vi "PicoScope6000AWG.vi"(6 "Arbitrary Waveform Settings":T1 {"Index Mode" items=["Single", "Dual", "Quad"]}, 7 "Standard Waveform Settings":T2 {"Start Frequency (Hz)" min=1 max=1000000}, 8 "error in":errorcluster, 9 "General AWG Settings":T3 {"White Noise/PRBS" items=["Normal", "White Noise", "PRBS"]; "Trigger Source" items=["None", "Scope Trigger", "Aux. In", "Ext. In", "Software Trigger"]; "Trigger Type" items=["Rising", "Falling", "Gate High", "Gate Low"]; "Sweep Type" items=["Up", "Down", "Up-Down", "Down-Up"]; "Wave Type" items=["Sine", "Square", "Triangle", "Ramp Up", "Ramp Down", "Sinc", "Gaussian", "Half Sine", "DC", "Arbitrary"]}, 11 "Handle In":i16) -> (0 "error out":errorcluster, 1 "Arbitrary\nWaveform Graph":i16[](graph), 2 "Trigger Source Out":u32, 3 "Handle Out":i16)   [LabVIEW 2009]
doc: "This VI can be used to control the arbitrary waveform generator. Standard waveforms can be selected or arbitrary waveform can be selected under 'Wave Type'. There are three settings clusters: general settings that apply to both arbitrary and standard waveforms, settings that apply only to standard waveforms and settings that apply only to arbitrary waveforms. It is not necessary to connect all of these clusters if only using arbitrary waveforms or only using standard waveforms are required.\n\nWhen selecting arbitrary waveform, it is necessary to specify a text file containing the wave form. This text file should have a single value on each line in the range -1 to 1. For further information on the settings, see descriptions of ps3000aSetSigGenBuiltIn and ps3000aSetSigGenArbitrary."
uses:
  ps6000.dll
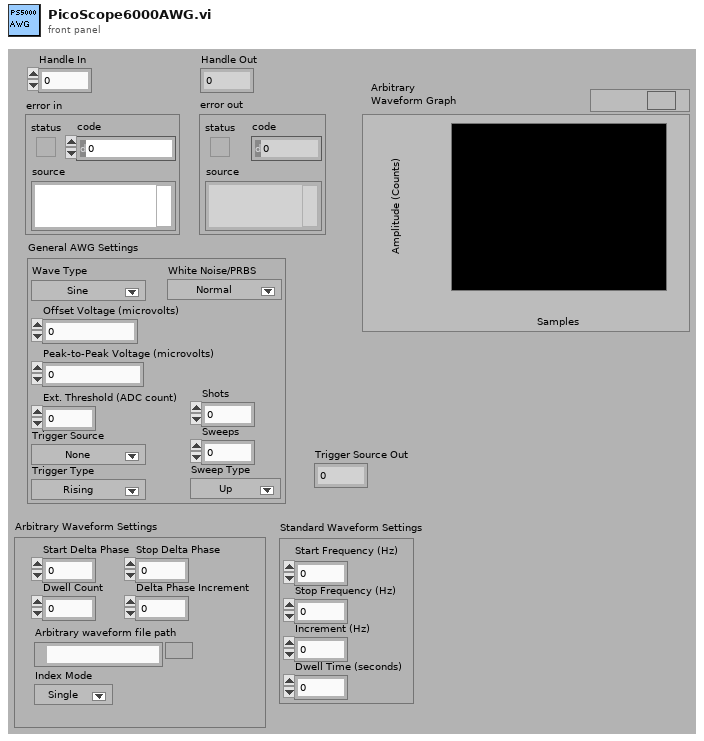
[diagram p1: front panel]
types:
  T1 = cluster{"Arbirary waveform file path":path, "Start Delta Phase":u32, "Index Mode":i32, "Stop Delta Phase":u32, "Delta Phase Increment":u32, "Dwell Count":u32}
  T2 = cluster{"Start Frequency (Hz)":sgl, "Stop Frequency (Hz)":sgl, "Increment (Hz)":sgl, "Dwell Time (seconds)":sgl}
  T3 = cluster{"Peak-to-Peak Voltage (microvolts)":u32, "Offset Voltage (microvolts)":i32, "Wave Type":u32, "Sweep Type":u32, "Shots":u32, "Sweeps":u32, "Trigger Type":u32, "Trigger Source":u32, "Ext. Threshold (ADC count)":i16, "White Noise/PRBS":u32}
  T4 = cluster{"status":bool, "code":u32, "source":string}
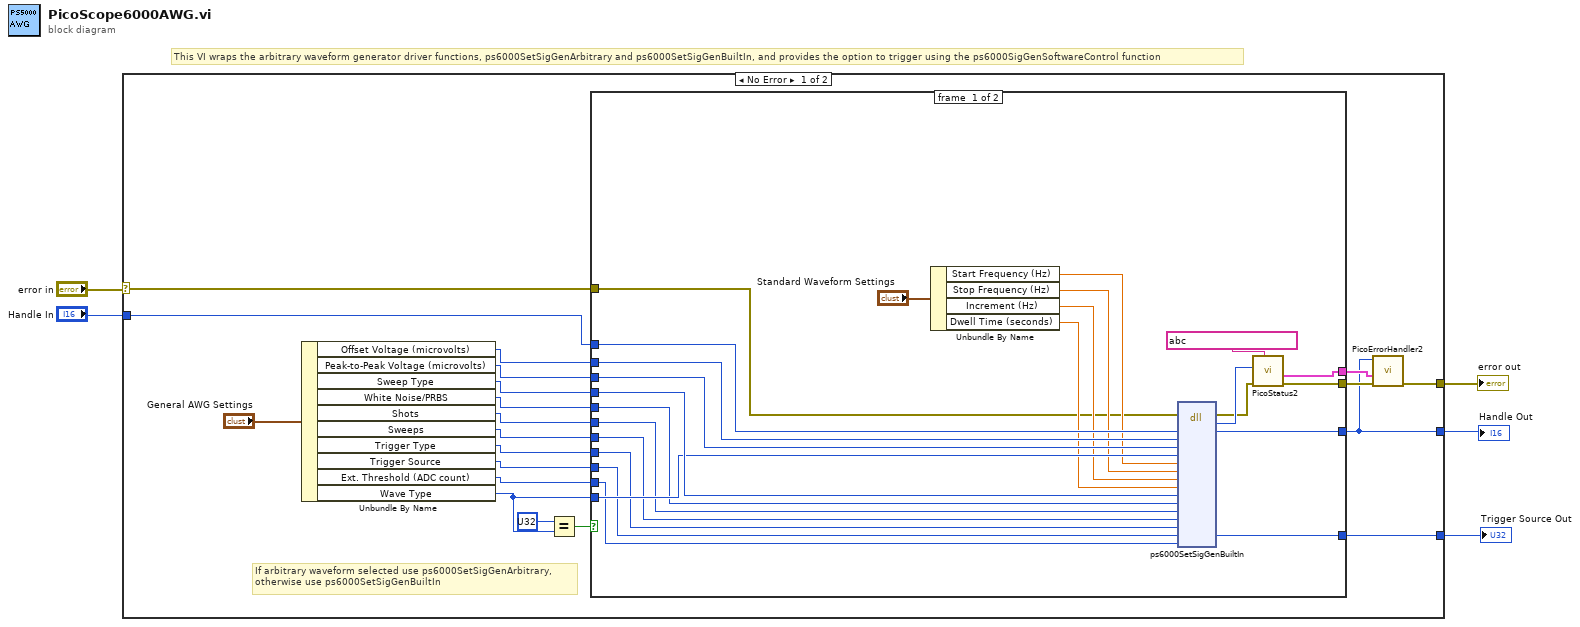
[diagram p0: block diagram]
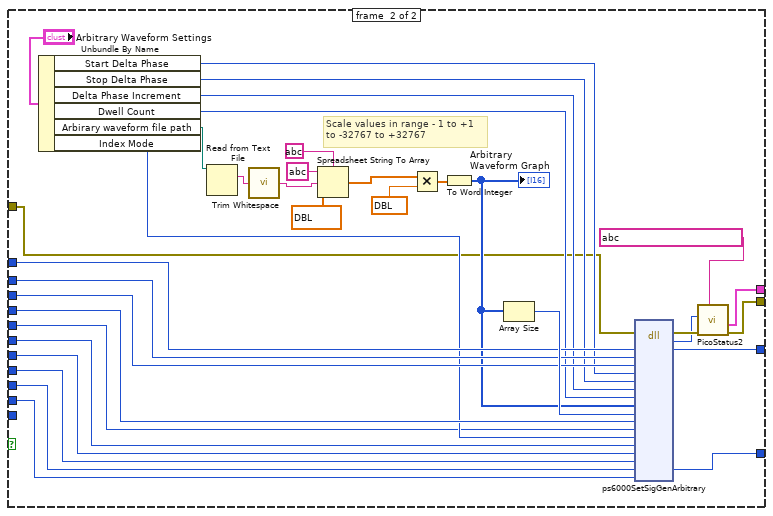
[diagram p2: hidden frame]
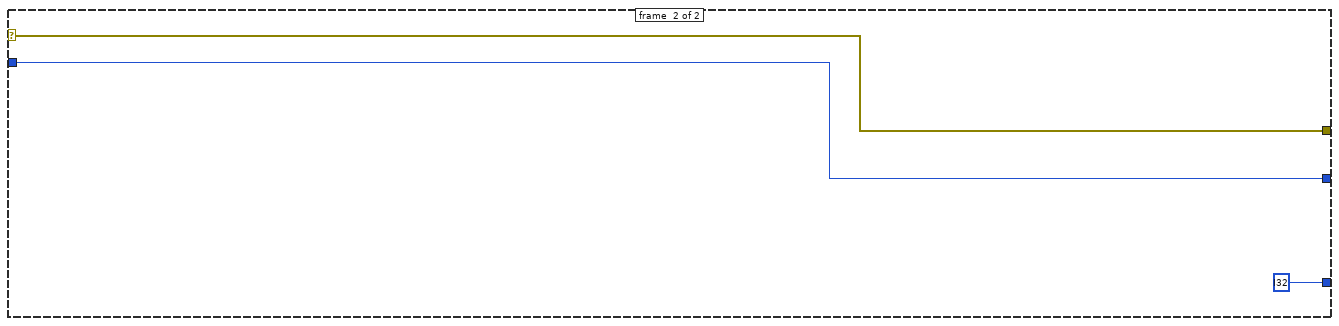
[diagram p3: hidden frame]
diagram:
  # "This VI wraps the arbitrary waveform generator driver functions, ps6000SetSigGenArbitrary and ps6000SetSigGenBuiltIn, and provides the option to trigger using the ps6000SigGenSoftwareControl function"
  n1 = case shown="No Error" "error in" {
    selector: "error in" -> [w11 w87]
    tunnel: [w6 w86] -> w5
    tunnel: "Handle In" -> [w23 w86]
    tunnel: [w8 w87] -> w3
    tunnel: [w10 i32 ?] -> w1
    frame #0 {
      # "If arbitrary waveform selected use ps6000SetSigGenArbitrary, \notherwise use ps6000SetSigGenBuiltIn"
      n2 = Unbundle By Name("General AWG Settings") -> ("Offset Voltage (microvolts)"=w21:i32, "Peak-to-Peak Voltage (microvolts)"=w20:u32, "Sweep Type"=w19:u32, "White Noise/PRBS"=w18:u32, "Shots"=w17:u32, "Sweeps"=w16:u32, "Trigger Type"=w15:u32, "Trigger Source"=w14:u32, "Ext. Threshold (ADC count)"=w13:i16, "Wave Type"=w12:u32)
      n3 = Equal?(x=u32 ?, y=w12) -> (x = y?=w25:bool)
      n4 = case shown="True" w25 {
        tunnel: [w49 w77] -> w6
        tunnel: w23 -> [w48 w78]
        tunnel: [w28 w52] -> w9
        tunnel: w21 -> [w47 w76]
        tunnel: w20 -> [w46 w75]
        tunnel: w19 -> [w45 w74]
        tunnel: w18 -> [w31 w57]
        tunnel: w17 -> [w43 w73]
        tunnel: w16 -> [w42 w72]
        tunnel: w15 -> [w41 w71]
        tunnel: w14 -> [w40 w70]
        tunnel: w13 -> [w39 w62]
        tunnel: w12 -> [w44 _]
        tunnel: [w33 w60] -> w10
        tunnel: w11 -> [w32 w59]
        tunnel: [w27 w50] -> w7
        frame #0 {
          n5 = Unbundle By Name("Standard Waveform Settings") -> ("Start Frequency (Hz)"=w37:sgl, "Stop Frequency (Hz)"=w36:sgl, "Increment (Hz)"=w35:sgl, "Dwell Time (seconds)"=w34:sgl)
          n6 = dll-call lib="ps6000.dll" fn="ps6000SetSigGenBuiltIn" ("ps3000.dll:_ps3000_open_unit@0")(error in=w32, "handle"=w48, "offsetVoltage"=w47, "pkToPk"=w46, "waveType"=w44, "startFrequency"=w37, "stopFrequency"=w36, "increment"=w35, "dwellTime"=w34, "sweepType"=w45, "operation"=w31, "shots"=w43, "sweeps"=w42, "triggerType"=w41, "triggerSource"=w40, "extInThreshold"=w39) -> (error out=w26:errorcluster, "PICO_STATUS"=w29:u32, "handle"=w49:i16, "triggerSource"=w33:u32)  [unwired: 15 in, 1 out]
          n7 = call "PicoStatus2.vi"("PICO source"=string ? ("source"), "Error in"=w26, "PICO STATUS"=w29) -> ("error out"=w28:errorcluster, "PICO_STATUS out"=w27:T4)  [unwired: 5 in]
        }
        frame #1 {
          # "Scale values in range - 1 to +1 \nto -32767 to +32767"
          n8 = Unbundle By Name("Arbitrary Waveform Settings") -> ("Start Delta Phase"=w68:u32, "Stop Delta Phase"=w67:u32, "Delta Phase Increment"=w65:u32, "Dwell Count"=w66:u32, "Arbirary waveform file path"=w64:path, "Index Mode"=w63:i32)
          n9 = Read from Text File(file (use dialog)=w64) -> (text=w56:string)  [unwired: 3 in, 3 out]
          n10 = call <vilib>:"Trim Whitespace.vi"("string"=w56) -> ("trimmed string"=w55:string)  [unwired: 1 in]
          n11 = Spreadsheet String To Array(delimiter (Tab)=string ?, format string=string ?, spreadsheet string=w55, array type (2D Dbl)=dbl[] ?) -> (array=w79:dbl[])
          n12 = Multiply(x=w79, y=dbl ? ("deltaPhaseIncrement")) -> (x*y=w58:dbl[])
          n13 = To Word Integer(number=w58) -> (16bit integer=w61:i16[])
          "Arbitrary\nWaveform Graph" <- w61
          n14 = Array Size(array=w61) -> (size(s)=w84:i32)
          n15 = dll-call lib="ps6000.dll" fn="ps6000SetSigGenArbitrary" ("ps3000.dll:_ps3000_open_unit@0")(error in=w59, "handle"=w78, "offsetVoltage"=w76, "pkToPk"=w75, "startDeltaPhase"=w68, "stopDeltaPhase"=w67, "deltaPhaseIncrement"=w65, "dwellCount"=w66, "arbitraryWaveform"=w61, "arbitraryWaveformSize"=w84, "sweepType"=w74, "operation"=w57, "indexMode"=w63, "shots"=w73, "sweeps"=w72, "triggerType"=w71, "triggerSource"=w70, "extInThreshold"=w62) -> (error out=w54:errorcluster, "PICO_STATUS"=w53:u32, "handle"=w77:i16, "triggerSource"=w60:u32)  [unwired: 17 in, 1 out]
          n16 = call "PicoStatus2.vi"("PICO source"=string ? ("source"), "Error in"=w54, "PICO STATUS"=w53) -> ("error out"=w52:errorcluster, "PICO_STATUS out"=w50:T4)  [unwired: 5 in]
        }
      }
      n17 = call "PicoErrorHandler2.vi"("error in (no error)"=w9, "PICO_STATUS in"=w7, "handle In"=w6) -> ("error out"=w8:errorcluster)  [unwired: 8 in]
    }
    frame #1 {
    }
  }
  "Handle Out" <- w5
  "error out" <- w3
  "Trigger Source Out" <- w1
